vi "Receive Interface Status.vi"(8 "error in (no error)":errorcluster, 11 "Stream in":refnum<class "Stream.lvclass">) -> (0 "error out":errorcluster, 3 "Stream out":refnum<class "Stream.lvclass">)   [LabVIEW 2018, in "Stream.lvclass"]
uses:
  Stream.lvclass
  Stream.lvclass/Stream.ctl
  Interface/Interface.lvclass
panel:
  out "STATUS":string
  out "COMMAND":string
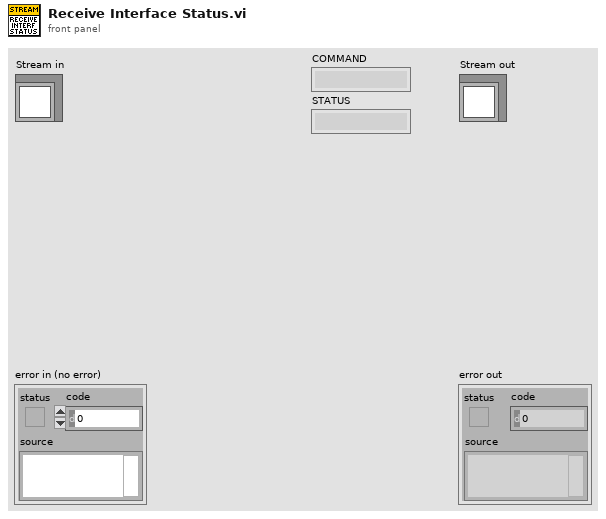
[diagram p1: front panel]
types:
  T1 = cluster{"Current Temperature":i16, "Temperatue Status":string}
  T2 = cluster{"Initialization":bool, "Serial Number":u16}
  T3 = cluster{"Exposure Time":sgl, "Pre-amp gain":u8, "Readout Rate":u8, "EM Mode":u8, "EM Gain":u16, "Binning":u16, "Initial Line":u16, "Initial Cloumn":u16, "Final Line":u16, "Final Column":u16, "Kinetic Series Length":u32, "Shutter Mode":u8, "Cooler ON/OFF":u16, "Temperature":i8, "Image Name":string, "Image Path":string, "#Images":u32, "#index":u16, "Trigger":u16}
  T4 = cluster{"Current Exptime":sgl, "Exposures Done":u16, "Last Image":string, "Disk Space":u16, "Exptime":sgl, "NImages":u16, "#index":u16, "File Base Name":string, "Image Path":string, "OBS Title":string, "Comment":string, "DS9":bool, "Cam_Status":string}
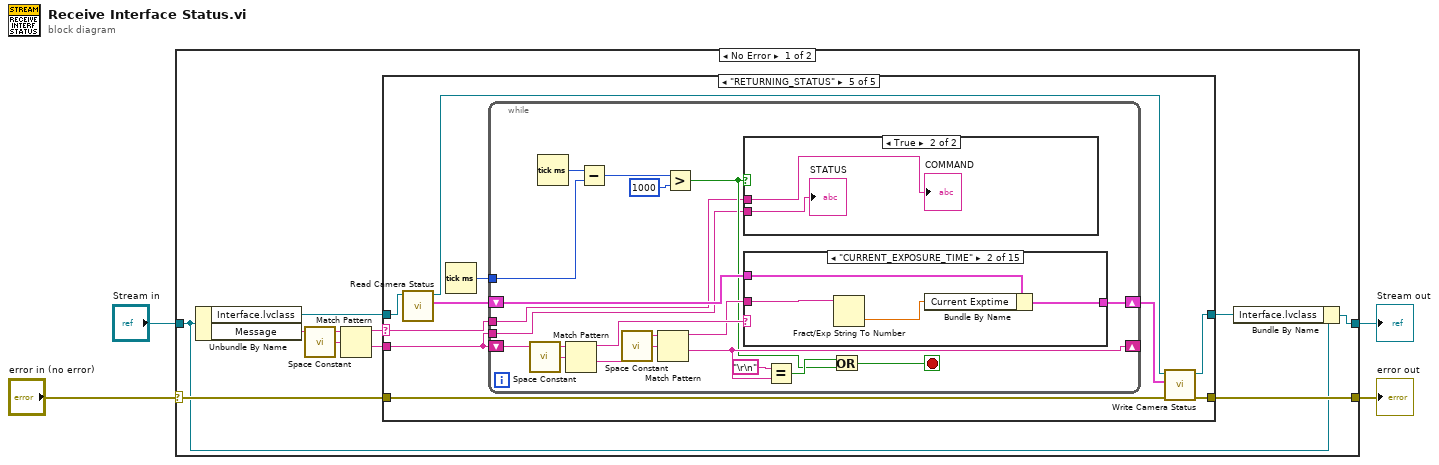
[diagram p0: block diagram]
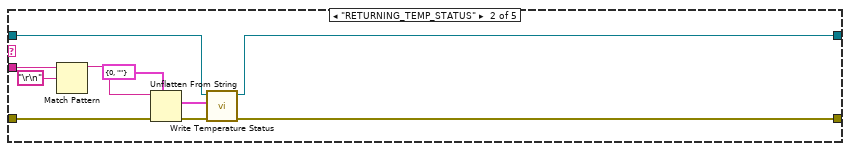
[diagram p3: hidden frame]
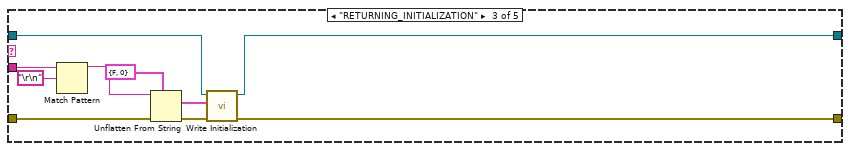
[diagram p4: hidden frame]
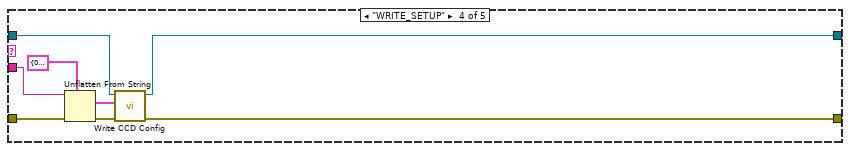
[diagram p5: hidden frame]
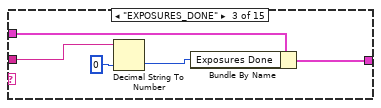
[diagram p8: hidden frame]
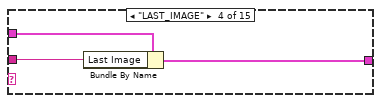
[diagram p9: hidden frame]
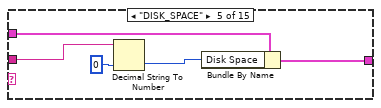
[diagram p10: hidden frame]
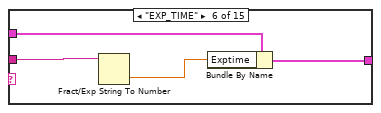
[diagram p11: hidden frame]
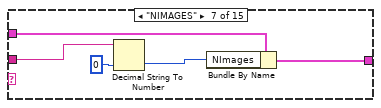
[diagram p12: hidden frame]
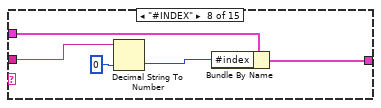
[diagram p13: hidden frame]
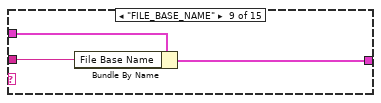
[diagram p14: hidden frame]
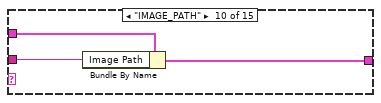
[diagram p15: hidden frame]
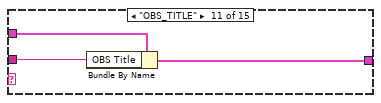
[diagram p16: hidden frame]
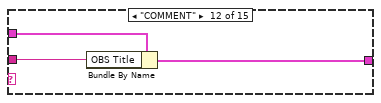
[diagram p17: hidden frame]
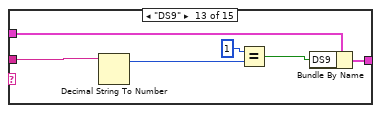
[diagram p18: hidden frame]
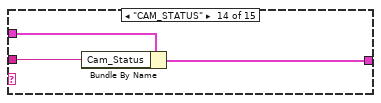
[diagram p19: hidden frame]
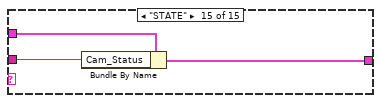
[diagram p20: hidden frame]
diagram:
  n1 = case shown="No Error" "error in (no error)" {
    selector: "error in (no error)" -> [w8 w133]
    tunnel: [w9 w133] -> w3
    tunnel: [w6 w132] -> w1
    tunnel: "Stream in" -> [w7 w132]
    frame No Error {
      n2 = Unbundle By Name(w7) -> ("Interface.lvclass"=w11:refnum<class "Interface.lvclass">, "Message"=w10:string)
      n3 = call <vilib>:"Space Constant.vi"() -> ("String"=w14:string)
      n4 = Match Pattern(string=w10, regular expression=w14) -> (before substring=w5:string, after substring=w13:string)  [unwired: 1 in, 2 out]
      n5 = case shown="\"RETURNING_STATUS\"" w5 {
        selector: w5 -> [_ _ _ _ w46]
        tunnel: w13 -> [_ w19 w28 w39 w45]
        tunnel: [w16 w26 w33 w41 w50] -> w12
        tunnel: w11 -> [w16 w25 w34 w40 w53]
        tunnel: [w15 w21 w32 w42 w49] -> w9
        tunnel: w8 -> [w15 w20 w31 w43 w48]
        frame "False", Default {
        }
        frame "RETURNING_TEMP_STATUS" {
          n6 = Match Pattern(string=w19, regular expression="\r\n") -> (before substring=w17:string)  [unwired: 1 in, 3 out]
          n7 = Unflatten From String(type=T1 {"Current Temperature"=0, "Temperatue Status"=""} ("Temperature Status"), binary string=w17, error in (no error)=w20) -> (value=w23:T1, error out=w24:errorcluster)  [unwired: 2 in, 1 out]
          n8 = call "Write Temperature Status.vi"("error in (no error)"=w24, "Temperature Status"=w23, "Interface in"=w25) -> ("error out"=w21:errorcluster, "Interface out"=w26:refnum<class "Interface.lvclass">)  [unwired: 7 in]
        }
        frame "RETURNING_INITIALIZATION" {
          n9 = Match Pattern(string=w28, regular expression="\r\n") -> (before substring=w27:string)  [unwired: 1 in, 3 out]
          n10 = Unflatten From String(type=T2 {"Initialization"=FALSE, "Serial Number"=0} ("Initialization"), binary string=w27, error in (no error)=w31) -> (value=w30:T2, error out=w36:errorcluster)  [unwired: 2 in, 1 out]
          n11 = call "Write Initialization.vi"("error in (no error)"=w36, "Initialization"=w30, "Interface in"=w34) -> ("error out"=w32:errorcluster, "Interface out"=w33:refnum<class "Interface.lvclass">)  [unwired: 7 in]
        }
        frame "WRITE_SETUP" {
          n12 = Unflatten From String(type=T3 {"Exposure Time"=0.0, "Pre-amp gain"=0, "Readout Rate"=0, "EM Mode"=0, "EM Gain"=0, "Binning"=0, "Initial Line"=0, "Initial Cloumn"=0, "Final Line"=0, "Final Column"=0, "Kinetic Series Length"=0, "Shutter Mode"=0, "Cooler ON/OFF"=0, "Temperature"=0, "Image Name"="", "Image Path"="", "#Images"=0, "#index"=0, "Trigger"=0} ("CCD Config"), binary string=w39, error in (no error)=w43) -> (value=w38:T3, error out=w44:errorcluster)  [unwired: 2 in, 1 out]
          n13 = call "Write CCD Config.vi"("error in (no error)"=w44, "CCD Config"=w38, "Interface in"=w40) -> ("error out"=w42:errorcluster, "Interface out"=w41:refnum<class "Interface.lvclass">)  [unwired: 7 in]
        }
        frame "RETURNING_STATUS" {
          n14 = call "Read Camera Status.vi"("Interface in"=w53) -> ("Camera Status"=w51:T4, "Interface out"=w52:refnum<class "Interface.lvclass">)  [unwired: 8 in, 1 out]
          n15 = Tick Count (ms)() -> (millisecond timer value=w47:u32)
          n16 = while {
            shift-right: [w70] -> w54
            shift-left: w51 -> [w69]
            shift-right: [w65] -> _
            shift-left: w45 -> [w72]
            tunnel: w47 -> [w62]
            tunnel: w46 -> [w56]
            tunnel: w45 -> [w55]
            stop <- w58 stop-if-true
            n17 = call <vilib>:"Space Constant.vi"() -> ("String"=w73:string)
            n18 = Tick Count (ms)() -> (millisecond timer value=w63:u32)
            n19 = Match Pattern(string=w72, regular expression=w73) -> (before substring=w71:string, after substring=w67:string)  [unwired: 1 in, 2 out]
            n20 = Subtract(x=w63, y=w62) -> (x-y=w61:u32)
            n21 = call <vilib>:"Space Constant.vi"() -> ("String"=w68:string)
            n22 = Match Pattern(string=w67, regular expression=w68) -> (before substring=w66:string, after substring=w65:string)  [unwired: 1 in, 2 out]
            n23 = Greater?(x=w61, y=1000) -> (0:w57:bool)
            n24 = case shown="True" w57 {
              tunnel: w56 -> [_ w75]
              tunnel: w55 -> [_ w74]
              frame False {
              }
              frame True {
                "COMMAND" <- w75
                "STATUS" <- w74
              }
            }
            n25 = case shown="\"CURRENT_EXPOSURE_TIME\"" w71 {
              tunnel: [w76 w80 w85 w88 w93 w97 w102 w107 w110 w113 w116 w119 w125 w128 w131] -> w70
              tunnel: w66 -> [_ w78 w83 w86 w90 w94 w99 w104 w108 w111 w114 w117 w123 w126 w129]
              tunnel: w69 -> [w76 w79 w84 w87 w92 w96 w101 w106 w109 w112 w115 w118 w124 w127 w130]
              frame "False", Default {
              }
              frame "CURRENT_EXPOSURE_TIME" {
                n26 = Fract/Exp String To Number(string=w78) -> (number=w77:dbl)  [unwired: 3 in, 1 out]
                n27 = Bundle By Name(cluster=w79, "Current Exptime"=w77) -> (w80:T4)
              }
              frame "EXPOSURES_DONE" {
                n28 = Decimal String To Number(string=w83, default (0L)=u16 0 ("default (0 I32)")) -> (number=w82:u16)  [unwired: 1 in, 1 out]
                n29 = Bundle By Name(cluster=w84, "Exposures Done"=w82) -> (w85:T4)
              }
              frame "LAST_IMAGE" {
                n30 = Bundle By Name(cluster=w87, "Last Image"=w86) -> (w88:T4)
              }
              frame "DISK_SPACE" {
                n31 = Decimal String To Number(string=w90, default (0L)=u16 0 ("default (0 I32)")) -> (number=w91:u16)  [unwired: 1 in, 1 out]
                n32 = Bundle By Name(cluster=w92, "Disk Space"=w91) -> (w93:T4)
              }
              frame "EXP_TIME" {
                n33 = Fract/Exp String To Number(string=w94) -> (number=w95:dbl)  [unwired: 3 in, 1 out]
                n34 = Bundle By Name(cluster=w96, "Exptime"=w95) -> (w97:T4)
              }
              frame "NIMAGES" {
                n35 = Decimal String To Number(string=w99, default (0L)=u16 0 ("default (0 I32)")) -> (number=w100:u16)  [unwired: 1 in, 1 out]
                n36 = Bundle By Name(cluster=w101, "NImages"=w100) -> (w102:T4)
              }
              frame "#INDEX" {
                n37 = Decimal String To Number(string=w104, default (0L)=u16 0 ("default (0 I32)")) -> (number=w105:u16)  [unwired: 1 in, 1 out]
                n38 = Bundle By Name(cluster=w106, "#index"=w105) -> (w107:T4)
              }
              frame "FILE_BASE_NAME" {
                n39 = Bundle By Name(cluster=w109, "File Base Name"=w108) -> (w110:T4)
              }
              frame "IMAGE_PATH" {
                n40 = Bundle By Name(cluster=w112, "Image Path"=w111) -> (w113:T4)
              }
              frame "OBS_TITLE" {
                n41 = Bundle By Name(cluster=w115, "OBS Title"=w114) -> (w116:T4)
              }
              frame "COMMENT" {
                n42 = Bundle By Name(cluster=w118, "OBS Title"=w117) -> (w119:T4)
              }
              frame "DS9" {
                n43 = Decimal String To Number(string=w123) -> (offset past number=w122:i32)  [unwired: 2 in, 1 out]
                n44 = Equal?(x=1, y=w122) -> (x = y?=w120:bool)
                n45 = Bundle By Name(cluster=w124, "DS9"=w120) -> (w125:T4)
              }
              frame "CAM_STATUS" {
                n46 = Bundle By Name(cluster=w127, "Cam_Status"=w126) -> (w128:T4)
              }
              frame "STATE" {
                n47 = Bundle By Name(cluster=w130, "Cam_Status"=w129) -> (w131:T4)
              }
            }
            n48 = Equal?(x="\r\n", y=w65) -> (x = y?=w59:bool)
            n49 = Or(x=w59, y=w57) -> (x .or. y?=w58:bool)
          }
          n50 = call "Write Camera Status.vi"("error in (no error)"=w48, "Camera Status"=w54, "Interface in"=w52) -> ("error out"=w49:errorcluster, "Interface out"=w50:refnum<class "Interface.lvclass">)  [unwired: 7 in]
        }
      }
      n51 = Bundle By Name(cluster=w7, "Interface.lvclass"=w12) -> (w6:refnum<class "Stream.lvclass">)
    }
    frame Error {
    }
  }
  "error out" <- w3
  "Stream out" <- w1
